vi "DAQ_Analog read.vi"(8 "error in (no error)":errorcluster, 11 "task/channels in":refnum<k21>="Photodetectors") -> (0 "error out":errorcluster, 2 "output cluster":T1)   [LabVIEW 2018]
uses:
  SupportVIs/DAQmx Read (Analog 1D DBL NChan 1Samp).vi
  SupportVIs/DAQmx Fill In Error Info.vi
  SupportVIs/NI_PtbyPt.lvlib
panel:
  out "Waveform Chart - Light":T2(graph)
  in  "stop":bool
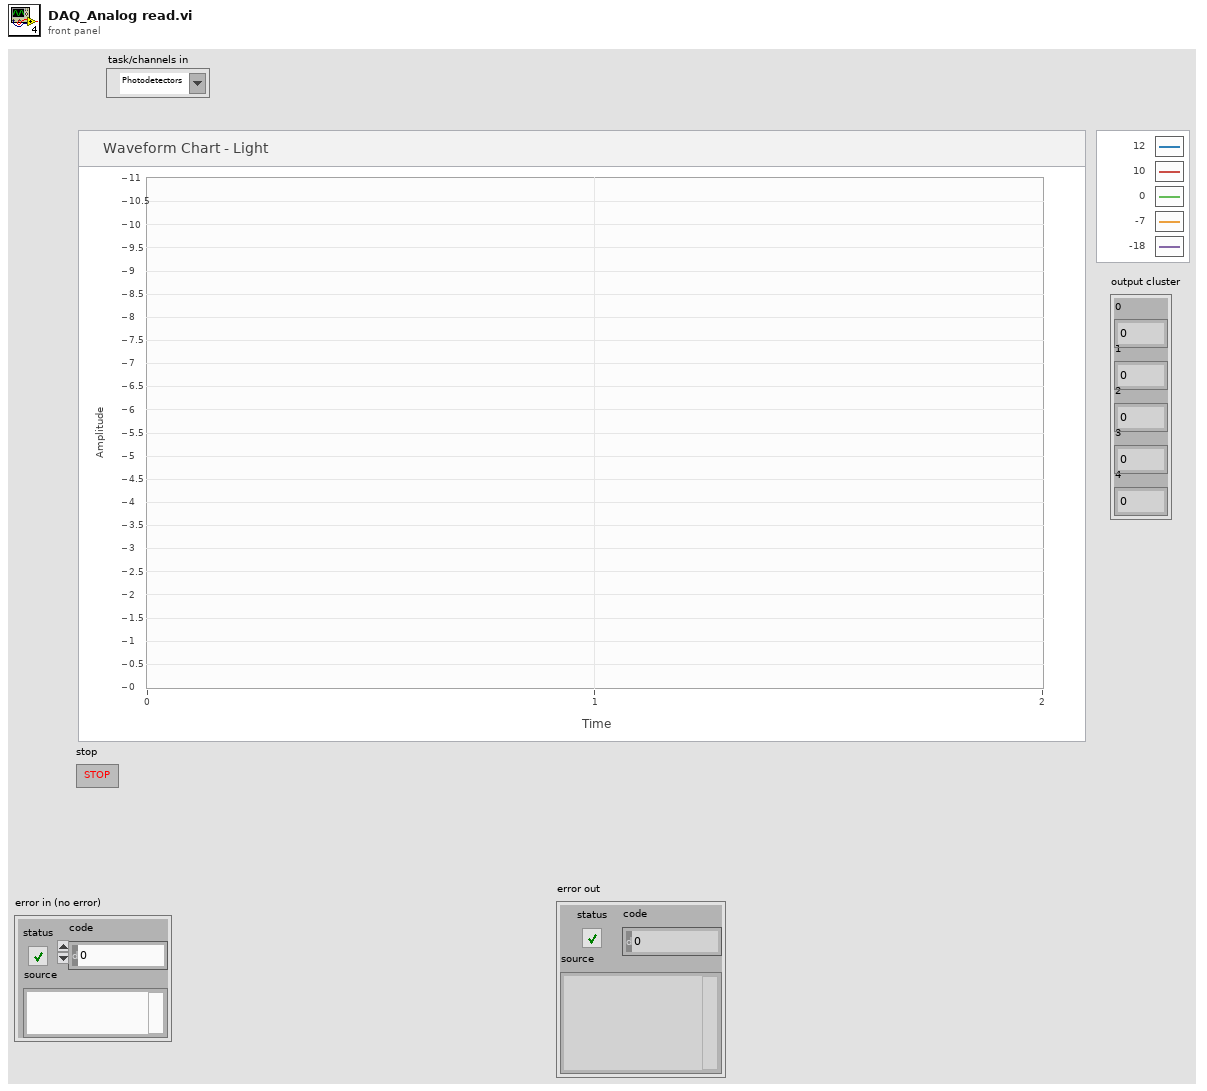
[diagram p1: front panel]
types:
  T1 = cluster{"0":dbl, "1":dbl, "2":dbl, "3":dbl, "4":dbl}
  T2 = cluster{"mean":dbl, "mean":dbl, "mean":dbl, "mean":dbl, "mean":dbl}
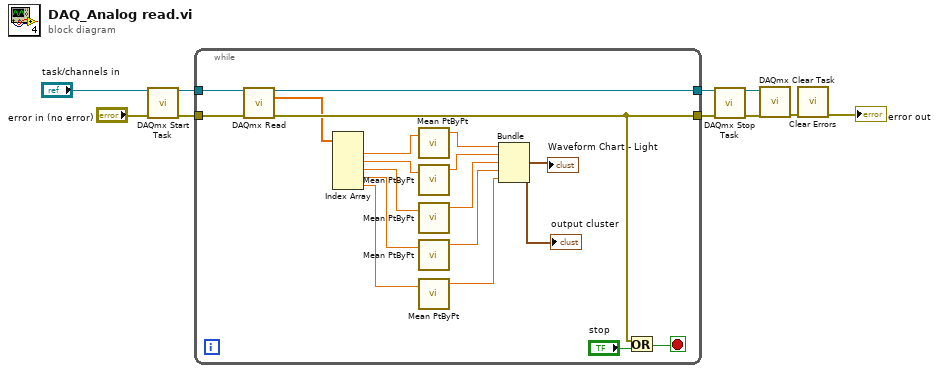
[diagram p0: block diagram]
diagram:
  n1 = call "DAQmx Start Task.vi"("task/channels in"="task/channels in", "error in"="error in (no error)") -> ("task out"=w10:refnum<k21>, "error out"=w9:errorcluster)  [unwired: 12 in]
  n2 = while {
    tunnel: w10 -> [w28]
    tunnel: w9 -> [w27]
    tunnel: [w25] -> w8
    tunnel: [w23] -> w7
    stop <- w24 stop-if-true
    n3 = call-poly "DAQmx Read.vi"("task/channels in"=w28, "error in"=w27) -> ("task out"=w25:refnum<k21>, "data"=w22:dbl[], "error out"=w23:errorcluster)  [unwired: 11 in]
    n4 = Index Array(array=w22) -> (element #1=w21:dbl, element #2=w19:dbl, element #3=w16:dbl, element #4=w15:dbl, element #5=w14:dbl)  [unwired: 5 in]
    n5 = call "Mean PtByPt.vi"("x"=w21) -> ("mean"=w20:dbl)  [unwired: 3 in, 1 out]
    n6 = call "Mean PtByPt.vi"("x"=w19) -> ("mean"=w18:dbl)  [unwired: 3 in, 1 out]
    n7 = call "Mean PtByPt.vi"("x"=w16) -> ("mean"=w13:dbl)  [unwired: 3 in, 1 out]
    n8 = call "Mean PtByPt.vi"("x"=w15) -> ("mean"=w12:dbl)  [unwired: 3 in, 1 out]
    n9 = call "Mean PtByPt.vi"("x"=w14) -> ("mean"=w11:dbl)  [unwired: 3 in, 1 out]
    n10 = Bundle("mean"=w20, "mean"=w18, "mean"=w13, "mean"=w12, "mean"=w11) -> (→"Waveform Chart - Light" →"output cluster":T2)  [unwired: 1 in]
    n11 = Or(x=w23, y="stop") -> (x .or. y?=w24:bool)
  }
  n12 = call "DAQmx Stop Task.vi"("task/channels in"=w8, "error in"=w7) -> ("task out"=w6:refnum<k21>, "error out"=w5:errorcluster)  [unwired: 12 in]
  n13 = call "DAQmx Clear Task.vi"("task in"=w6, "error in"=w5) -> ("error out"=w4:errorcluster)  [unwired: 13 in]
  n14 = call "Clear Errors.vi"("error in (no error)"=w4) -> ("error out"=→"error out":errorcluster)  [unwired: 5 in, 1 out]
